vi "CTRE_Phoenix_CANcoder_SetPosition.vi"(6 "timeoutMs":u32, 8 "error in (no error)":errorcluster, 10 "Position":dbl, 11 "CTRE_CANcoder_DeviceRef":T1) -> (0 "error out":errorcluster, 3 "CTRE_CANcoder_DeviceRef":T1)   [LabVIEW 2019]
doc: "Sets the position of the sensor. The units are determined by the coefficient and unit-string configuration params, default is degrees."
uses:
  <vilib>/Rock Robotics/WPI/ThirdParty/Phoenix-LabVIEW/CANCoder/Controls/CTRE_Phoenix_CANcoder_DeviceRef.ctl
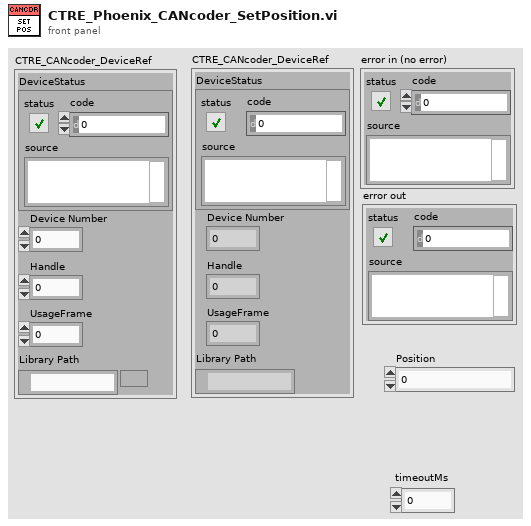
[diagram p1: front panel]
types:
  T1 = typedef "CTRE_Phoenix_CANcoder_DeviceRef.ctl" = cluster{"DeviceStatus":errorcluster, "Device Number":u8, "Handle":u64, "UsageFrame":u32, "Library Path":path}
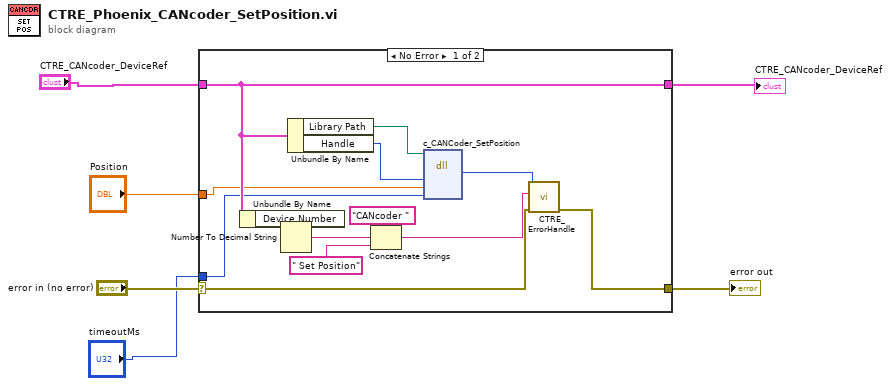
[diagram p0: block diagram]
diagram:
  n1 = case shown="No Error" "error in (no error)" {
    selector: "error in (no error)" -> [w10 w20]
    tunnel: [w9 w20] -> w5
    tunnel: [w12 w21] -> w1
    tunnel: "CTRE_CANcoder_DeviceRef" -> [w12 w21]
    tunnel: "Position" -> [w8 _]
    tunnel: "timeoutMs" -> [w7 _]
    frame No Error {
      n2 = Unbundle By Name(w12) -> ("Device Number"=w16:u8)
      n3 = Number To Decimal String(number=w16) -> (decimal integer string=w15:string)  [unwired: 1 in]
      n4 = Unbundle By Name(w12) -> ("Library Path"=w19:path, "Handle"=w18:u64)
      n5 = Concatenate Strings("CANcoder " ("string"), w15, " Set Position" ("string")) -> (w11:string)
      n6 = dll-call lib="?" fn="c_CANCoder_SetPosition"(path in=w19, "handle"=w18, "position"=w8, "timeoutms"=w7) -> ("return type"=w17:i32)  [unwired: 5 in, 2 out]
      n7 = call <vilib>:"CTRE_ErrorHandle.vi"("error in"=w10, "origin"=w11, "code"=w17) -> ("error out"=w9:errorcluster)  [unwired: 8 in]
    }
    frame Error {
    }
  }
  "error out" <- w5
  "CTRE_CANcoder_DeviceRef" <- w1
